vi "GetDeviceData.vi"(11 "ID":string) -> (1 "Type 2":string, 2 "DB Serial Number 2":string, 3 "ID 2":string, 5 "?":bool)   [LabVIEW 2019]
panel:
  in  "?":bool
  in  "Type":string
  in  "DB Serial Number":string
  out "?":string
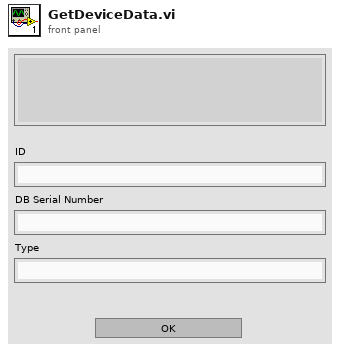
[diagram p1: front panel]
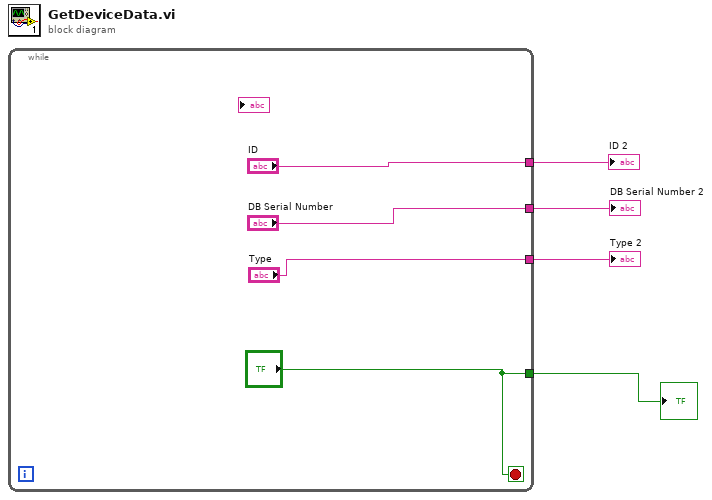
[diagram p0: block diagram]
diagram:
  n1 = while {
    tunnel: ["ID"] -> w4
    tunnel: ["DB Serial Number"] -> w3
    tunnel: ["Type"] -> w2
    tunnel: ["?"] -> w1
    stop <- "?" stop-if-true
  }
  "ID 2" <- w4
  "DB Serial Number 2" <- w3
  "Type 2" <- w2
  "?" <- w1
